vi "Configure Discrete Sweep (Custom).vi"(0 "template configuration":refnum<class "SV Signal.lvclass">, 5 "custom list":T1(array[cluster]) {"amplitude [V]" format="%.2f"; "frequency [Hz]" format="%.2f"}, 11 "error in (no error)":errorcluster) -> (4 "signal configuration":refnum<class "SV Discrete Sweep.lvclass">, 15 "error out":errorcluster)   [LabVIEW 2017, in "SV Discrete Sweep.lvclass"]
doc: "Configures a user-defined test signal. Wire the outputs to SV Signal (waveform) VI to generate the test signal, or wire to SV Signal Property Node to configure additional parameters before wiring to the SV Signal (waveform) VI."
uses:
  <vilib>/addons/_NISVFA/_Generation/Signal Generation/SV Discrete Sweep/SV Discrete Sweep.lvclass
  C:/Program Files (x86)/National Instruments/LabVIEW 2017/vi.lib/addons/_NISVFA/_Generation/Signal Generation/SV Function/SV Function.lvclass
  C:/Program Files (x86)/National Instruments/LabVIEW 2017/vi.lib/addons/_NISVFA/_Generation/Signal Generation/SV Signal/SV Signal.lvclass
  <vilib>/addons/_NISVFA/_Generation/Signal Generation/SV Signal/SV Signal.lvclass
  <vilib>/addons/_NISVFA/_Generation/Signal Generation/SV Signal/sv_System Timing Model.ctl
  <vilib>/addons/_NISVFA/_Generation/Signal Generation/SV Discrete Sweep/SV Discrete Sweep.lvclass/SV Discrete Sweep.ctl
  <vilib>/addons/_NISVFA/_Generation/Signal Generation/SV Signal/Write System Timing Model.vi
  <vilib>/addons/_NISVFA/_Generation/Signal Generation/SV Function/Write Measurement Cycles.vi
  <vilib>/addons/_NISVFA/_Generation/Signal Generation/SV Signal/Write Sample Rate.vi
  <vilib>/addons/_NISVFA/_Generation/Signal Generation/SV Function/SV Function.lvclass
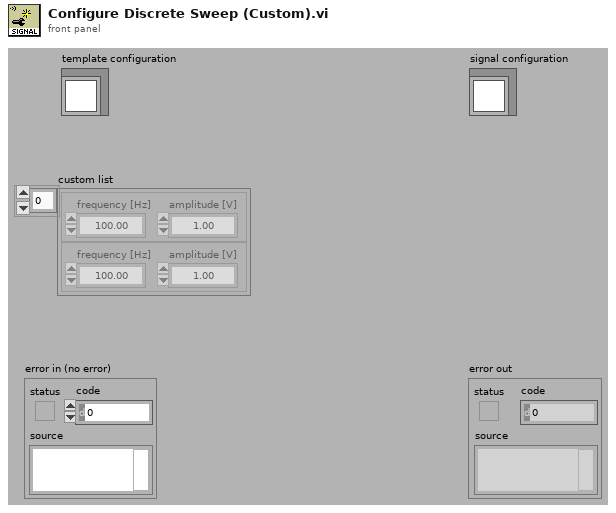
[diagram p1: front panel]
types:
  T1 = cluster{"frequency [Hz]":dbl, "amplitude [V]":dbl}[]
  T2 = typedef "SV Signal.lvclass/sv_System Timing Model.ctl" = i64
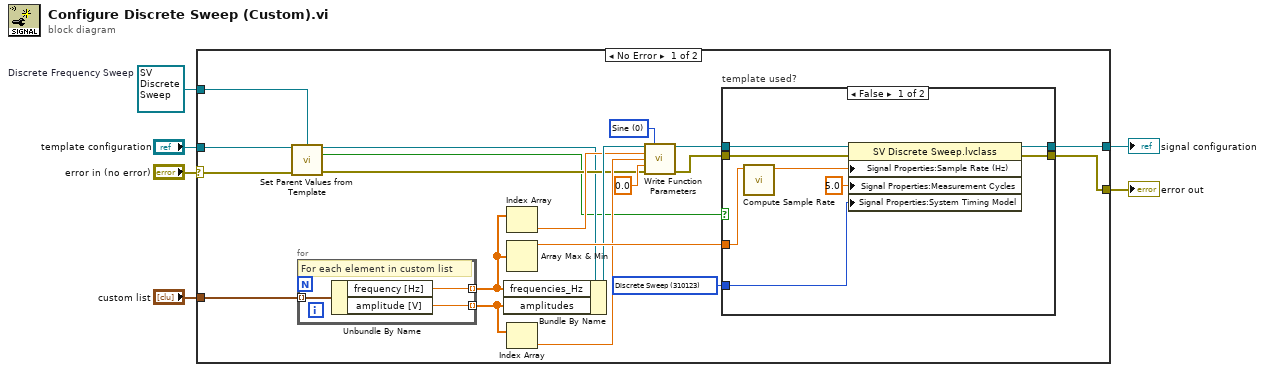
[diagram p0: block diagram]
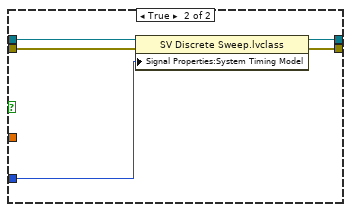
[diagram p2: hidden frame]
diagram:
  w4 = refnum<class "SV Discrete Sweep.lvclass"> refnum  # Discrete Frequency Sweep
  n1 = case shown="No Error" "error in (no error)" {
    selector: "error in (no error)" -> [w11 w43]
    tunnel: [w23 w43] -> w5
    tunnel: [w26 w44] -> w3
    tunnel: w4 -> [w8 w44]
    tunnel: "custom list" -> [w19 _]
    tunnel: "template configuration" -> [w12 _]
    frame No Error {
      w15 = u16 0 items=["Sine", "Triangle", "Square", "Sawtooth"] ("function type")
      w24 = T2 310123 items=["Finite"=10178, "-"=-1, "Continuous"=10123, "-"=-2, "Settled"=110123, "Averaged"=210123, "Discrete Sweep"=310123, "Continuous Sweep"=410123] ("System Timing Model")
      n2 = call-dynamic "Set Parent Values from Template.vi"("template configuration"=w12, "signal configuration in"=w8, "error in (no error)"=w11) -> ("signal configuration out"=w9:refnum<class "SV Discrete Sweep.lvclass">, "template used?"=w7:bool, "error out"=w10:errorcluster)  [unwired: 10 in]
      n3 = for {
        tunnel: w19 -> [w42] mode=indexing
        tunnel: [w41] -> w18 mode=indexing
        tunnel: [w40] -> w17 mode=indexing
        # "For each element in custom list"
        n4 = Unbundle By Name(w42) -> ("frequency [Hz]"=w41:dbl, "amplitude [V]"=w40:dbl)
      }
      n5 = Bundle By Name(cluster=w9, "frequencies_Hz"=w18, "amplitudes"=w17) -> (w22:refnum<class "SV Discrete Sweep.lvclass">)
      n6 = Index Array(array=w18) -> (element=w16:dbl)  [unwired: 1 in]
      n7 = Array Max & Min(array=w18) -> (max value=w25:dbl)  [unwired: 3 out]
      n8 = Index Array(array=w17) -> (element=w14:dbl)  [unwired: 1 in]
      n9 = call <vilib>:"Write Function Parameters.vi"("signal configuration"=w22, "function type"=w15, "frequency (Hz)"=w16, "amplitude"=w14, "phase (deg)"=0.0, "error in (no error)"=w10) -> ("signal configuration"=w21:refnum<class "SV Discrete Sweep.lvclass">, "error out"=w20:errorcluster)  [unwired: 8 in]
      n10 = case "template used?" shown="False" w7 {
        tunnel: [w33 w39] -> w26
        tunnel: w25 -> [w32 _]
        tunnel: w24 -> [w30 w38]
        tunnel: [w29 w37] -> w23
        tunnel: w21 -> [w28 w36]
        tunnel: w20 -> [w27 w35]
        frame False {
          n11 = call <vilib>:"Compute Sample Rate.vi"("maximum frequency [Hz]"=w32) -> ("sample rate [Hz]"=w31:dbl)  [unwired: 10 in]
          n12 = property class="SV Discrete Sweep.lvclass"(reference=w28, error in=w27, "Signal Properties:Sample Rate (Hz)"=w31, "Signal Properties:Measurement Cycles"=5.0 ("Measurement Cycles"), "Signal Properties:System Timing Model"=w30) -> (reference out=w33:refnum<class "SV Discrete Sweep.lvclass">, error out=w29:errorcluster)
        }
        frame True {
          n13 = property class="SV Discrete Sweep.lvclass"(reference=w36, error in=w35, "Signal Properties:System Timing Model"=w38) -> (reference out=w39:refnum<class "SV Discrete Sweep.lvclass">, error out=w37:errorcluster)
        }
      }
    }
    frame Error {
    }
  }
  "error out" <- w5
  "signal configuration" <- w3
